vi "PulseTrainGenerator-Single.vi"(8 "Stop Button":bool) -> ()   [LabVIEW 2015]
panel:
  out "error?":bool
  in  "Ch Setup":T1={"IP Address"="192.168.126.147", "DIO #"=0, "Frequency (Hz)"=100.0, "duty cycle (%)"=0.5, "Enable"=FALSE} {"duty cycle (%)" min=0.01 max=0.99 step=0.1; "Frequency (Hz)" min=0.0 step=10.0}
  in  "Startup Index":u16
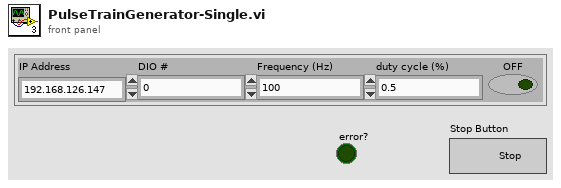
[diagram p1: front panel]
types:
  T1 = cluster{"IP Address":string, "DIO #":u16, "Frequency (Hz)":dbl, "duty cycle (%)":dbl, "Enable":bool}
  T2 = enum16{"Enable", "Disable", "Change Frequency", "Change Duty Cycle", "Configure", "Configure and Run"}
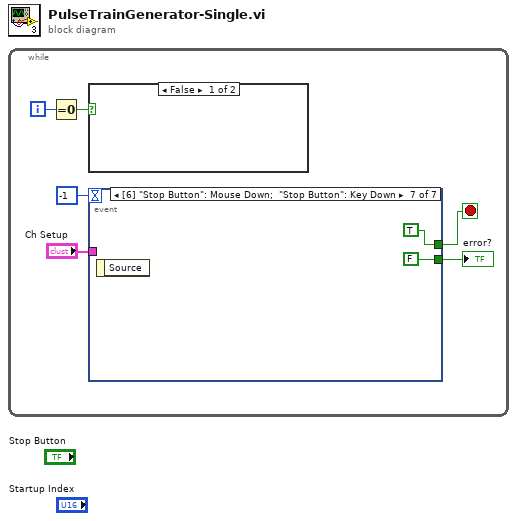
[diagram p0: block diagram]
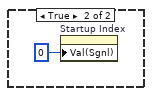
[diagram p2: hidden frame]
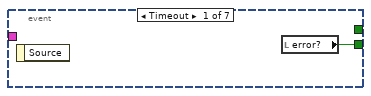
[diagram p3: hidden frame]
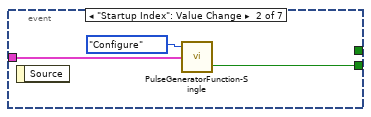
[diagram p4: hidden frame]
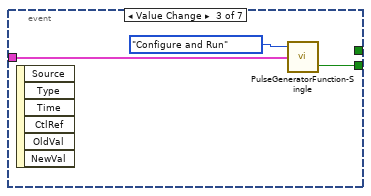
[diagram p5: hidden frame]
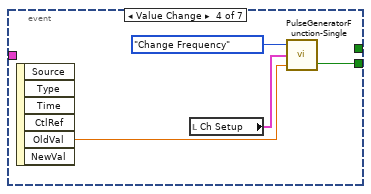
[diagram p6: hidden frame]
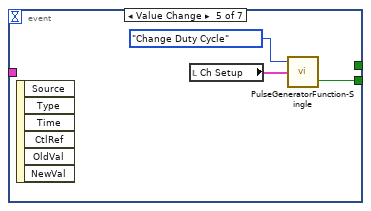
[diagram p7: hidden frame]
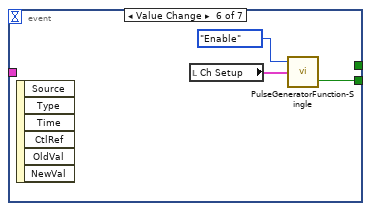
[diagram p8: hidden frame]
diagram:
  n1 = while {
    i -> [w6]
    stop <- w4 stop-if-true
    n2 = Equal To 0?(x=w6) -> (x = 0?=w5:bool)
    n3 = case shown="False" w5 {
      frame False {
      }
      frame True {
        n4 = property on="Startup Index" class="DigNum (strict)"("Val(Sgnl)"=u16 0 ("Value (Signaling)")) -> ()  [unwired: 2 in, 2 out]
      }
    }
    n5 = event shown="[6] \"Stop Button\": Mouse Down;  \"Stop Button\": Key Down" {
      selector: _ -> [_ _ _ _ _ _ _]
      dyn-events: _ -> [_ _ _ _ _ _ _]
      timeout: -1 -> [_ _ _ _ _ _ _]
      tunnel: "Ch Setup" -> [_ w11 w14 _ _ _ _]
      tunnel: [_ _ _ _ _ _ TRUE] -> w4
      tunnel: [w8 w9 w12 w16 w19 w22 FALSE ("error?")] -> w2
      event Timeout {
        n6 = event-data() -> ()  [unwired: 1 in, 1 out]
        n7 = local read "error?"() -> (w8:bool)
      }
      event "Startup Index": Value Change {
        n8 = event-data() -> ()  [unwired: 1 in, 1 out]
        n9 = call "PulseGeneratorFunction-Single.vi"("Ch Setup"=w11, "Mode"=T2."Configure") -> ("error?"=w9:bool)  [unwired: 2 in]
      }
      event "Ch Setup.IP Address", "Ch Setup.DIO #": Value Change {
        n10 = event-data() -> ()  [unwired: 1 in, 6 out]
        n11 = call "PulseGeneratorFunction-Single.vi"("Ch Setup"=w14, "Mode"=T2."Configure and Run") -> ("error?"=w12:bool)  [unwired: 2 in]
      }
      event "Ch Setup.Frequency (Hz)": Value Change {
        n12 = event-data() -> ("OldVal"=w15:dbl)  [unwired: 1 in, 5 out]
        n13 = local read "Ch Setup"() -> (w18:T1)
        n14 = call "PulseGeneratorFunction-Single.vi"("Frequency_old (Hz)"=w15, "Ch Setup"=w18, "Mode"=T2."Change Frequency") -> ("error?"=w16:bool)  [unwired: 1 in]
      }
      event "Ch Setup.duty cycle (%)": Value Change {
        n15 = event-data() -> ()  [unwired: 1 in, 6 out]
        n16 = local read "Ch Setup"() -> (w21:T1)
        n17 = call "PulseGeneratorFunction-Single.vi"("Ch Setup"=w21, "Mode"=T2."Change Duty Cycle") -> ("error?"=w19:bool)  [unwired: 2 in]
      }
      event "Ch Setup.Enable": Value Change {
        n18 = event-data() -> ()  [unwired: 1 in, 6 out]
        n19 = local read "Ch Setup"() -> (w24:T1)
        n20 = call "PulseGeneratorFunction-Single.vi"("Ch Setup"=w24, "Mode"=T2."Enable") -> ("error?"=w22:bool)  [unwired: 2 in]
      }
      event "Stop Button": Mouse Down; "Stop Button": Key Down {
        n21 = event-data() -> ()  [unwired: 1 in, 1 out]
      }
    }
    "error?" <- w2
  }
